vi "Digital Output.vi"(8 "error in":errorcluster, 11 "DAQmx Task Name":refnum<k21>) -> (0 "error out":errorcluster, 3 "DAQmx Task Name Out":refnum<k21>)   [LabVIEW 2021]
uses:
  <vilib>/DAQmx/write.llb/DAQmx Write (Digital 1D Bool 1Chan 1Samp).vi
  <vilib>/DAQmx/miscellaneous.llb/DAQmx Fill In Error Info.vi
  <resource>/objmgr/daqmx.rc
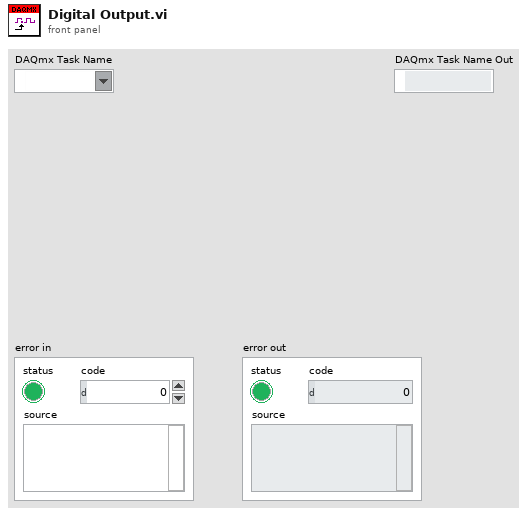
[diagram p1: front panel]
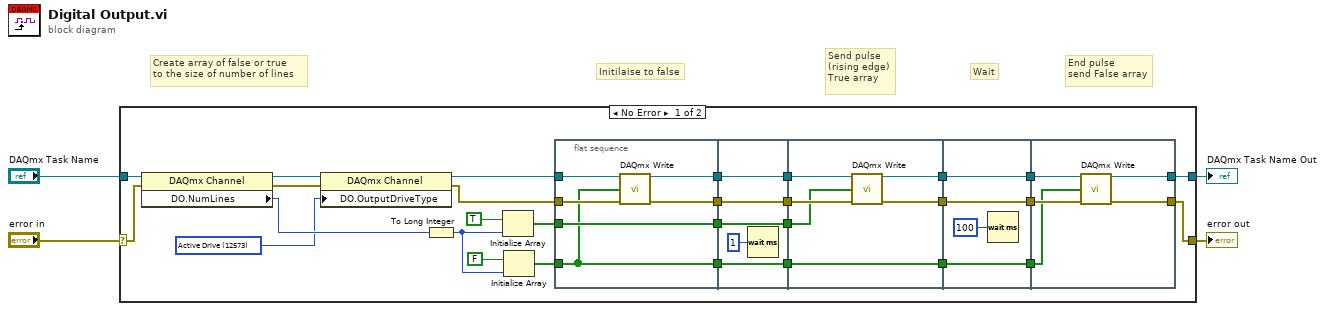
[diagram p0: block diagram]
diagram:
  # "End pulse\nsend False array"
  # "Wait"
  # "Send pulse\n(rising edge)\nTrue array"
  # "Initilaise to false"
  # "Create array of false or true\nto the size of number of lines"
  n1 = case shown="No Error" "error in" {
    selector: "error in" -> [w10 w61]
    tunnel: [w11 w61] -> w1
    tunnel: "DAQmx Task Name" -> [w28 w60]
    tunnel: [w29 w60] -> w2
    frame No Error {
      w5 = 12573 items=["Active Drive"=12573, "Open Collector"=12574] ("DO.OutputDriveType")
      n2 = property class="DAQmx Channel"(reference=w28, error in=w10) -> (reference out=w6:refnum<k21>, error out=w9:errorcluster, "DO.NumLines"=w26:u32)
      n3 = property class="DAQmx Channel"(reference=w6, error in=w9, "DO.OutputDriveType"=w5) -> (reference out=w7:refnum<k21>, error out=w8:errorcluster)
      n4 = To Long Integer(number=w26) -> (32bit integer=w24:i32)
      n5 = Initialize Array(TRUE, w24) -> (w25:bool[])
      n6 = Initialize Array(FALSE, w24) -> (w22:bool[])
      n7 = flat-sequence {
        tunnel: w22 -> [w34]
        tunnel: w25 -> [w39]
        tunnel: [w39] -> w15
        tunnel: [w34] -> w14
        tunnel: w7 -> [w38]
        tunnel: [w37] -> w13
        tunnel: w8 -> [w36]
        tunnel: [w35] -> w12
        tunnel: [w41] -> w19
        tunnel: [w40] -> w18
        tunnel: [w44] -> w17
        tunnel: [w43] -> w16
        tunnel: w15 -> [w44]
        tunnel: w14 -> [w43]
        tunnel: w13 -> [w41]
        tunnel: w12 -> [w40]
        tunnel: [w48] -> w33
        tunnel: [w47] -> w32
        tunnel: [w45] -> w21
        tunnel: w19 -> [w50]
        tunnel: w18 -> [w49]
        tunnel: w17 -> [w46]
        tunnel: w16 -> [w45]
        tunnel: w33 -> [w54]
        tunnel: w32 -> [w53]
        tunnel: [w54] -> w31
        tunnel: [w53] -> w30
        tunnel: w21 -> [w51]
        tunnel: [w51] -> w20
        tunnel: [w58] -> w29
        tunnel: [w56] -> w11
        tunnel: w31 -> [w57]
        tunnel: w30 -> [w59]
        tunnel: w20 -> [w55]
        frame #0 {
          n8 = call-poly <vilib>:"DAQmx Write.vi"("task/channels in"=w38, "data"=w34, "error in"=w36) -> ("task out"=w37:refnum<k21>, "error out"=w35:errorcluster)  [unwired: 10 in, 1 out]
        }
        frame #1 {
          n9 = Wait (ms)(milliseconds to wait=u32 1) -> ()  [unwired: 1 out]
        }
        frame #2 {
          n10 = call-poly <vilib>:"DAQmx Write.vi"("task/channels in"=w50, "data"=w46, "error in"=w49) -> ("task out"=w47:refnum<k21>, "error out"=w48:errorcluster)  [unwired: 10 in, 1 out]
        }
        frame #3 {
          n11 = Wait (ms)(milliseconds to wait=u32 100) -> ()  [unwired: 1 out]
        }
        frame #4 {
          n12 = call-poly <vilib>:"DAQmx Write.vi"("task/channels in"=w59, "data"=w55, "error in"=w57) -> ("task out"=w58:refnum<k21>, "error out"=w56:errorcluster)  [unwired: 10 in, 1 out]
        }
      }
    }
    frame Error {
    }
  }
  "error out" <- w1
  "DAQmx Task Name Out" <- w2
